vi "SetVIRefnum.vi"(8 "error in (no error)":errorcluster, 10 "VI Refnum":refnum<vi>, 11 "object in":refnum<class "Vi_Button.lvclass">) -> (0 "error out":errorcluster, 3 "object out":refnum<class "Vi_Button.lvclass">)   [LabVIEW 2012, in "Vi_Button.lvclass"]
uses:
  Vi_Button.lvclass
  Vi_Button.lvclass/Vi_Button.ctl
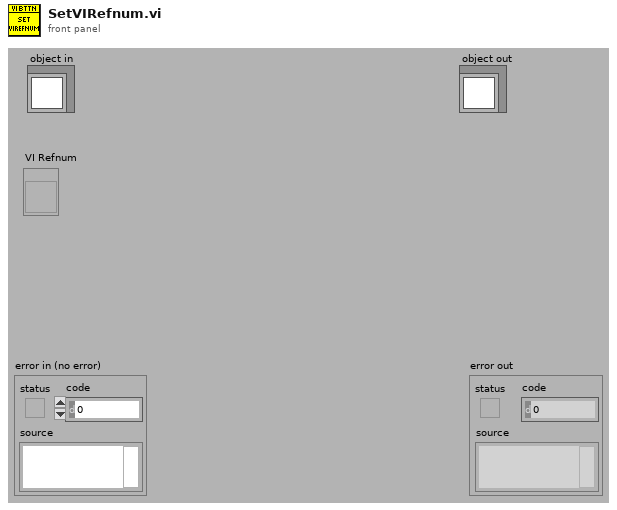
[diagram p1: front panel]
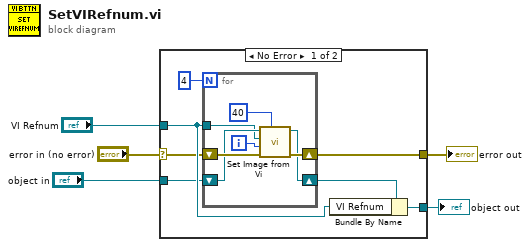
[diagram p0: block diagram]
diagram:
  n1 = case shown="No Error" "error in (no error)" {
    selector: "error in (no error)" -> [w10 w21]
    tunnel: [w9 w21] -> w4
    tunnel: [w12 w20] -> w2
    tunnel: "object in" -> [w8 w20]
    tunnel: "VI Refnum" -> [w11 _]
    frame No Error {
      n2 = for {
        N: 4 -> [_]
        shift-right: [w17] -> w7
        shift-left: w8 -> [w16]
        shift-right: [w18] -> w9
        shift-left: w10 -> [w19]
        tunnel: w11 -> [w14]
        i -> [w13]
        n3 = call-dynamic "Set Image from Vi.vi"("Button Size"=40, "error in (no error)"=w19, "State"=w13, "VI Refnum"=w14, "Button in"=w16) -> ("error out"=w18:errorcluster, "Button out"=w17:refnum<class "Vi_Button.lvclass">)  [unwired: 1 in, 4 out]
      }
      n4 = Bundle By Name(cluster=w7, "VI Refnum"=w11) -> (w12:refnum<class "Vi_Button.lvclass">)
    }
    frame Error {
    }
  }
  "error out" <- w4
  "object out" <- w2
